vi "Make Command Tag from Name.vi"(10 "Time":dbl, 11 "Cmd Name":string="%.3f secs") -> (3 "Cmd Tag":string)   [LabVIEW 2025]
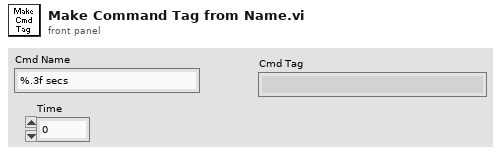
[diagram p1: front panel]
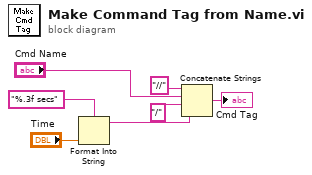
[diagram p0: block diagram]
diagram:
  n1 = Format Into String(format string="%.3f secs", "Time") -> (resulting string=w3:string)  [unwired: 2 in, 1 out]
  n2 = Concatenate Strings("//", "Cmd Name", "/", w3) -> (→"Cmd Tag":string)
